vi "Test Case, Wake-Up.vi"() -> ()   [LabVIEW 2010]
panel:
  out "error out":errorcluster
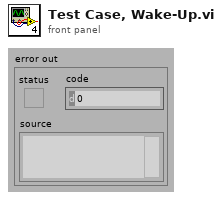
[diagram p1: front panel]
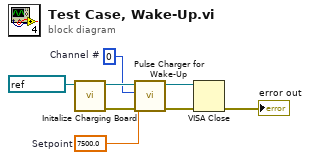
[diagram p0: block diagram]
diagram:
  w1 = 7500.0  # Setpoint
  w2 = 0  # Channel #
  n1 = call "Initalize Charging Board.vi"("VISA resource (Charging Board)"=refnum<visa-resource-name> "COM8") -> ("error out"=w6:errorcluster, "VISA resource out"=w4:refnum<visa-resource-name>)  [unwired: 9 in]
  n2 = call "Pulse Charger for Wake-Up.vi"("error in"=w6, "Setpoint"=w1, "Channel #"=w2, "VISA resource (Charging Board)"=w4) -> ("error out"=w5:errorcluster, "VISA resource (Charging Board) dup"=w3:refnum<visa-resource-name>)  [unwired: 6 in]
  n3 = VISA Close(VISA resource name=w3, error in (no error)=w5) -> (error out=→"error out":errorcluster)
